vi "Start.vi"(8 "error in (no error)":errorcluster, 10 "Message in":refnum<class "StartMessage.lvclass">, 11 "DAQCascade512 in":refnum<class "DAQCascade512.lvclass">) -> (0 "error out":errorcluster, 3 "DAQCascade512 out":refnum<class "DAQCascade512.lvclass">)   [LabVIEW 2012, in "DAQCascade512.lvclass"]
doc: "This member function is called when the statemachine in the run.vi receives an 'start' command. It relays the message to all observers of the component.\n\nOverride this member function in your derived class if you need additional start functionality (but don't forget to call the parent method)."
uses:
  DAQCascade512.lvclass
  <vilib>/Distrio/Murmex/StartMessage/StartMessage.lvclass
  <vilib>/Distrio/Murmex/Murmex/Murmex.lvclass
  DAQCascade512.lvclass/DAQCascade512.ctl
panel:
  in  "stop":bool=TRUE
  out "img":sgl[][](graph)
  out "Data type":u32
  out "No. of images":i32=10
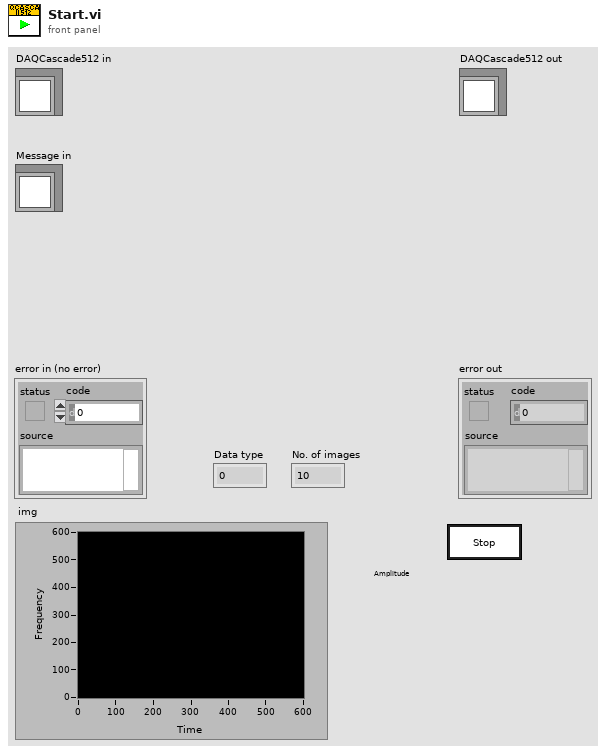
[diagram p1: front panel]
types:
  T1 = typedef "Image_type.ctl" = u32
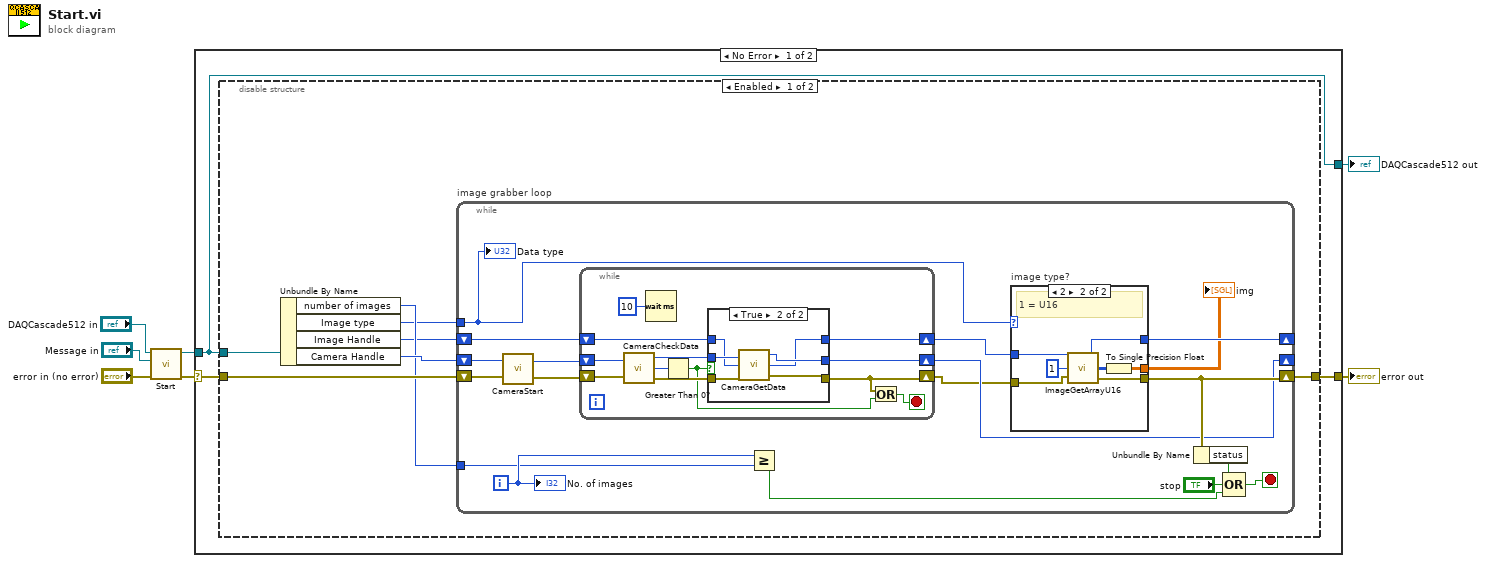
[diagram p0: block diagram]
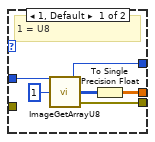
[diagram p3: hidden frame]
diagram:
  n1 = call-parent "Start.vi"("error in (no error)"="error in (no error)", "Message in"="Message in", "Murmex in"="DAQCascade512 in") -> ("error out"=w2:errorcluster, "Murmex out"=w4:refnum<class "DAQCascade512.lvclass">)  [unwired: 7 in]
  n2 = case shown="No Error" w2 {
    selector: w2 -> [w9 w72]
    tunnel: w4 -> [w8 w71]
    tunnel: [w10 w72] -> w3
    tunnel: [w8 w71] -> w1
    frame No Error {
      n3 = disable-structure shown="Enabled" {
        disable-tunnel: [w17 w70] -> w10
        disable-tunnel: w9 -> [w14 w70]
        disable-tunnel: w8 -> [w16 _]
        frame Enabled {
          n4 = Unbundle By Name(w16) -> ("number of images"=w13:u32, "Image type"=w12:T1, "Image Handle"=w11:u32, "Camera Handle"=w15:u32)
          n5 = while "image grabber loop" {
            shift-right: [w34] -> _
            shift-left: w11 -> [w18]
            shift-right: [w25] -> _
            shift-left: w15 -> [w22]
            shift-right: [w35] -> w17
            shift-left: w14 -> [w23]
            tunnel: w12 -> [w19]
            tunnel: w13 -> [w28]
            i -> [w29]
            stop <- w32 stop-if-true
            n6 = call <userlib>:"CameraStart.vi"("error in"=w23, "Camera Handle"=w22) -> ("error out"=w20:errorcluster, "Camera Handle"=w21:u32)
            n7 = while {
              shift-right: [w42] -> w25
              shift-left: w21 -> [w46]
              shift-right: [w40] -> w26
              shift-left: w18 -> [w41]
              shift-right: [w38] -> w24
              shift-left: w20 -> [w47]
              stop <- w39 stop-if-true
              n8 = call <userlib>:"CameraCheckData.vi"("Camera Handle"=w46, "error in"=w47) -> ("Camera Handle"=w43:u32, "Number Of Frames Available"=w45:i32, "error out"=w44:errorcluster)
              n9 = Wait (ms)(milliseconds to wait=u32 10) -> ()  [unwired: 1 out]
              n10 = Greater Than 0?(x=w45) -> (x > 0?=w37:bool)
              n11 = case shown="True" w37 {
                tunnel: w44 -> [w49 w56]
                tunnel: w43 -> [w50 w55]
                tunnel: [w50 w54] -> w42
                tunnel: [w49 w53] -> w38
                tunnel: w41 -> [w48 w52]
                tunnel: [w48 w51] -> w40
                frame False {
                }
                frame True {
                  n12 = call <userlib>:"CameraGetData.vi"("error in"=w56, "Data Handle"=w52, "Camera Handle"=w55) -> ("error out"=w53:errorcluster, "Data Handle"=w51:u32, "Camera Handle"=w54:u32)
                }
              }
              n13 = Or(x=w38, y=w37) -> (x .or. y?=w39:bool)
            }
            n14 = Greater Or Equal?(x=w29, y=w28) -> (x >= y?=w27:bool)
            n15 = case "image type?" shown="2" w19 {
              tunnel: [w62 w69] -> w35
              tunnel: [w61 w68] -> w34
              tunnel: [w58 w64] -> w30
              tunnel: w26 -> [w59 w66]
              tunnel: w24 -> [_ w63]
              frame 1, Default {
                # "1 = U8"
                n16 = call <userlib>:"ImageGetArrayU8.vi"("Z Position"=u32 1, "Image Handle"=w59) -> ("error out"=w62:errorcluster, "Array"=w60:u8[][], "Image Handle"=w61:u32)  [unwired: 1 in]
                n17 = To Single Precision Float(number=w60) -> (single precision float=w58:sgl[][])
              }
              frame 2 {
                # "1 = U16"
                n18 = call <userlib>:"ImageGetArrayU16.vi"("error in"=w63, "Z position"=u32 1, "Image Handle"=w66) -> ("error out"=w69:errorcluster, "Array uint 16"=w67:u16[][], "Image Handle"=w68:u32)
                n19 = To Single Precision Float(number=w67) -> (single precision float=w64:sgl[][])
              }
            }
            "img" <- w30
            n20 = Unbundle By Name(w35) -> ("status"=w33:bool)
            n21 = Compound Arithmetic op=OR(w33, "stop", w27) -> (w32:bool)
            "Data type" <- w19
            "No. of images" <- w29
          }
        }
        frame Disabled {
        }
      }
    }
    frame Error {
    }
  }
  "error out" <- w3
  "DAQCascade512 out" <- w1
